vi "flow-NTR.vi"() -> (3 "NTR Flow":T1[](array[typedef]))   [LabVIEW 2024]
uses:
  controls/UiStepBuilder.ctl
  controls/type.step-builder.ctl
  globals/globals-engine.vi
panel:
  in  "Cycle Interval [s]":u16
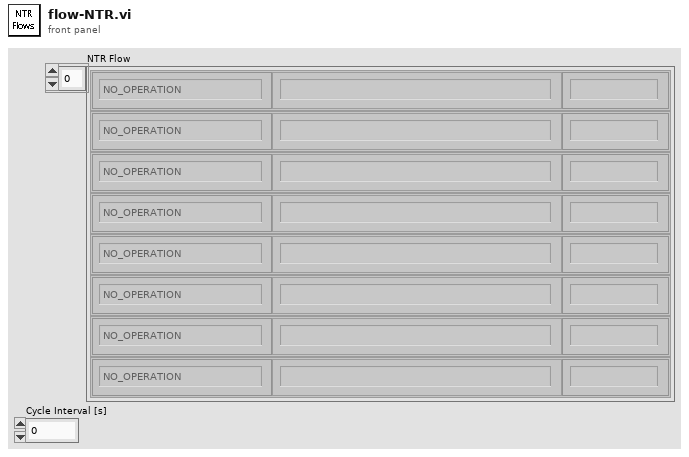
[diagram p1: front panel]
types:
  T1 = typedef "UiStepBuilder.ctl" = cluster{"Step Function":T2, "ParamString":string, "Step Label":string}
  T2 = typedef "type.step-builder.ctl" = enum16{"NO_OPERATION", "DELAY-JUMP", "DELAY", "JUMP", "COMPLETE", "SCHEDULER", "IRR-CHECK", "UNIT-CHECK", "UNIT-SAMPLE", "UNIT-DOSE", "LOG-REPORT", "LOG-MESSAGE", "IO-READ", "IO-READ-MANY", "IO-WRITE", "IO-COMPARE-OUT", "IO-COMPARE-IN", "PROC-START", "PROC-STOP", "PROC-LOAD", "PROC-IS-COMPLETED", "RECORD-MOVE", "GET-RH", "GET-UV", "GET-WD", "GET-WS", "OCS-CHECK", "OCS-RECORD"}
  T3 = typedef "UiNutritionPanel.ctl" = cluster{"Main":cluster{"Enable":bool, "WashTimes":cluster{"In":dbl, "Out":dbl}, "DailyActivityHours":cluster{"Begin Time":T4, "End Time":T4}[]}, "Water Dosing":cluster{"Water Dose":dbl, "Water Limit":dbl}, "EC Ranges":cluster{"H Alarm":dbl, "L Alarm":dbl, "Low":dbl}, "EC Dosing":cluster{"ALFA1 Dose":dbl, "ALFA1 Limit":dbl, "BETA1 Dose":dbl, "BETA1 Limit":dbl, "ALFA2 Dose":dbl, "ALFA2 Limit":dbl, "BETA2 Dose":dbl, "BETA2 Limit":dbl}, "PH Ranges":cluster{"H Alarm":dbl, "L Alarm":dbl, "High":dbl, "Low":dbl}, "PH Dosing":cluster{"ACID Dose":dbl, "ACID Limit":dbl, "BASE Dose":dbl, "BASE Limit":dbl}, "ORP Ranges":cluster{"H Alarm":dbl, "L Alarm":dbl, "Low":dbl}, "ORP Dosing":cluster{"MIX Dose":dbl, "MIX Limit":dbl}}
  T4 = typedef "UiScheduleTimestamp.ctl" = timestamp
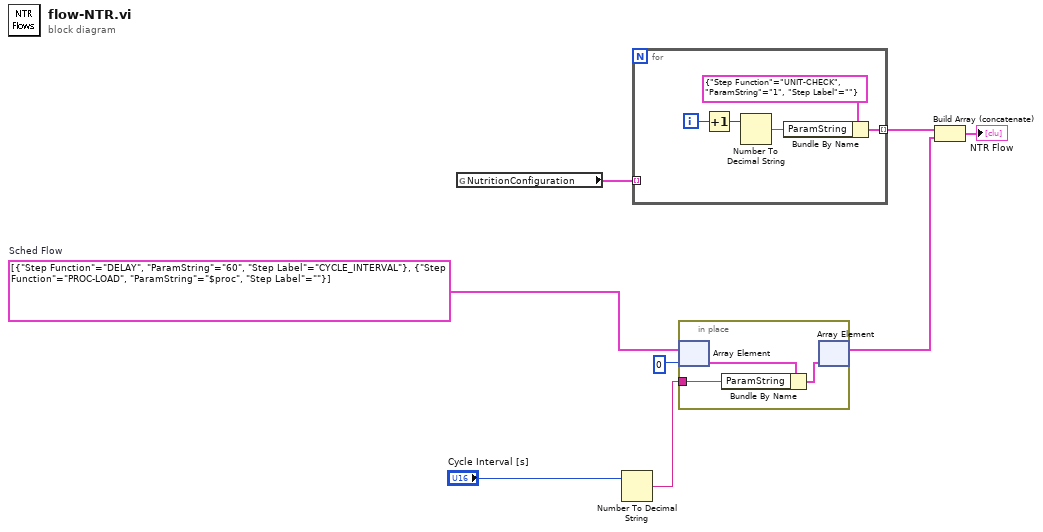
[diagram p0: block diagram]
diagram:
  w3 = T1[] [{"Step Function"=enum."DELAY", "ParamString"="60", "Step Label"="CYCLE_INTERVAL"}, {"Step Function"=enum."PROC-LOAD", "ParamString"="$proc", "Step Label"=""}]  # Sched Flow
  n1 = global read "globals-engine.vi" "NutritionConfiguration"() -> (w1:T3[])
  n2 = Number To Decimal String(number="Cycle Interval [s]") -> (decimal integer string=w5:string)  [unwired: 1 in]
  n3 = for {
    tunnel: w1 -> [_] mode=indexing
    tunnel: [w9] -> w7 mode=indexing
    i -> [w12]
    n4 = Increment(x=w12) -> (x+1=w10:i32)
    n5 = Number To Decimal String(number=w10) -> (decimal integer string=w11:string)  [unwired: 1 in]
    n6 = Bundle By Name(cluster=T1 {"Step Function"=enum."UNIT-CHECK", "ParamString"="1", "Step Label"=""} ("UiBuilderStep"), "ParamString"=w11) -> (w9:T1)
  }
  n7 = in-place {
    in-place-border: w5 -> [w15]
    n8 = in-place-array #1(w3, 0) -> (w16:T1)
    n9 = Bundle By Name(cluster=w16, "ParamString"=w15) -> (w14:T1)
    n10 = in-place-array #1(w14) -> (w2:T1[])  [unwired: 1 out]
  }
  n11 = Build Array (concatenate)(w7, w2) -> (→"NTR Flow":T1[])
